vi "SetupCalc.vi"(8 "error in (no error)":errorcluster caption="entrée d'erreur (pas d'erreur)", 9 "Experiment.lvclass":refnum<class "Experiment.lvclass">=refnum, 11 "Interface en entrée":refnum<class "Interface.lvclass"> caption="Interface Class in") -> (0 "error out":errorcluster caption="sortie d'erreur", 1 "Experiment.lvclass Out":refnum<class "Experiment.lvclass">, 3 "Interface en sortie":refnum<class "Interface.lvclass"> caption="Interface Class out")   [LabVIEW 2019, in "Interface.lvclass"]
uses:
  Interface.lvclass
  Experiment Class/Experiment.lvclass
  DevicesClass/Tools/Tools.lvclass
  Calculations Class/DefaultDev_Func.ctl
  CurveSetup.ctl
  DevicesClass/BaseDevice/BaseDevice.lvclass
  Calculations Class/Calculations.lvclass
  C:/Programmes Labview/LabscanV1A/DevicesClass/BaseDevice/BaseDevice.lvclass
  Interface.lvclass/Interface.ctl
  Experiment Class/Experiment.lvclass/Experiment.ctl
  Calculations Class/Calculations.lvclass/Calculations.ctl
  DevicesClass/BaseDevice/BaseDevice.lvclass/BaseDevice.ctl
  Calculations Class/Accessor/GetOperation Name.vi
  Experiment Class/Accessor/GetLoadedTools.vi
  DevicesClass/BaseDevice/Accessor/SetClassEvent.vi
  DevicesClass/BaseDevice/Accessor/SetClassQueue.vi
  Experiment Class/Accessor/SetLoadedTools.vi
  DevicesClass/BaseDevice/Accessor/GetClassEvent.vi
  DevicesClass/BaseDevice/Accessor/GetClassQueue.vi
panel:
  out "InstrClassEventQ":T1(array[cluster])
  out "Edit Mode":bool
  out "ToolIndex":i32
  in  "Save Par":bool
  in  "EditOper":bool
  out "LoadedTools":refnum<class "BaseDevice.lvclass">[](array[class])
  in  "OperationName":string
  out "PanelViRefOut":refnum<vi>[](array[refnum])
  out "Y Values":dbl[](array[numeric])
  out "X Values":dbl[](array[numeric])
  in  "ScanDatSrc":bool[](array[boolean])
  in  "RemOper":bool
  in  "RemDataSrc":bool
  in  "Created Calc":i32(listbox) caption="Created calculation"
  in  "Data Source":i32(listbox) caption="Calculation Data Source"
  in  "AddAqData":bool
  in  "Acquired Data List":i32(listbox)
  out "2D Scan":bool
  in  "2D Plot Act":bool caption="2D Plot"
  in  "Data Only":bool
  in  "AddDataSrc":bool
  out "GraphIndex":i32
  in  "CreateOper":bool
  in  "DisplayName":string
  out "CrvParOut":T2[](array[typedef])
  out "NomDon":string[](array[string])=["RTêta;", "X&Y;"]
  out "VarParams":string[][](array[string])
  in  "ScanParam":u16(ring) caption="Scan Parameter" items=["Tools.Ind Point(Point)", "Tools_0"]
  in  "Operation":T3
  in  "stop":bool
  in  "Scan Data List":i32(listbox)
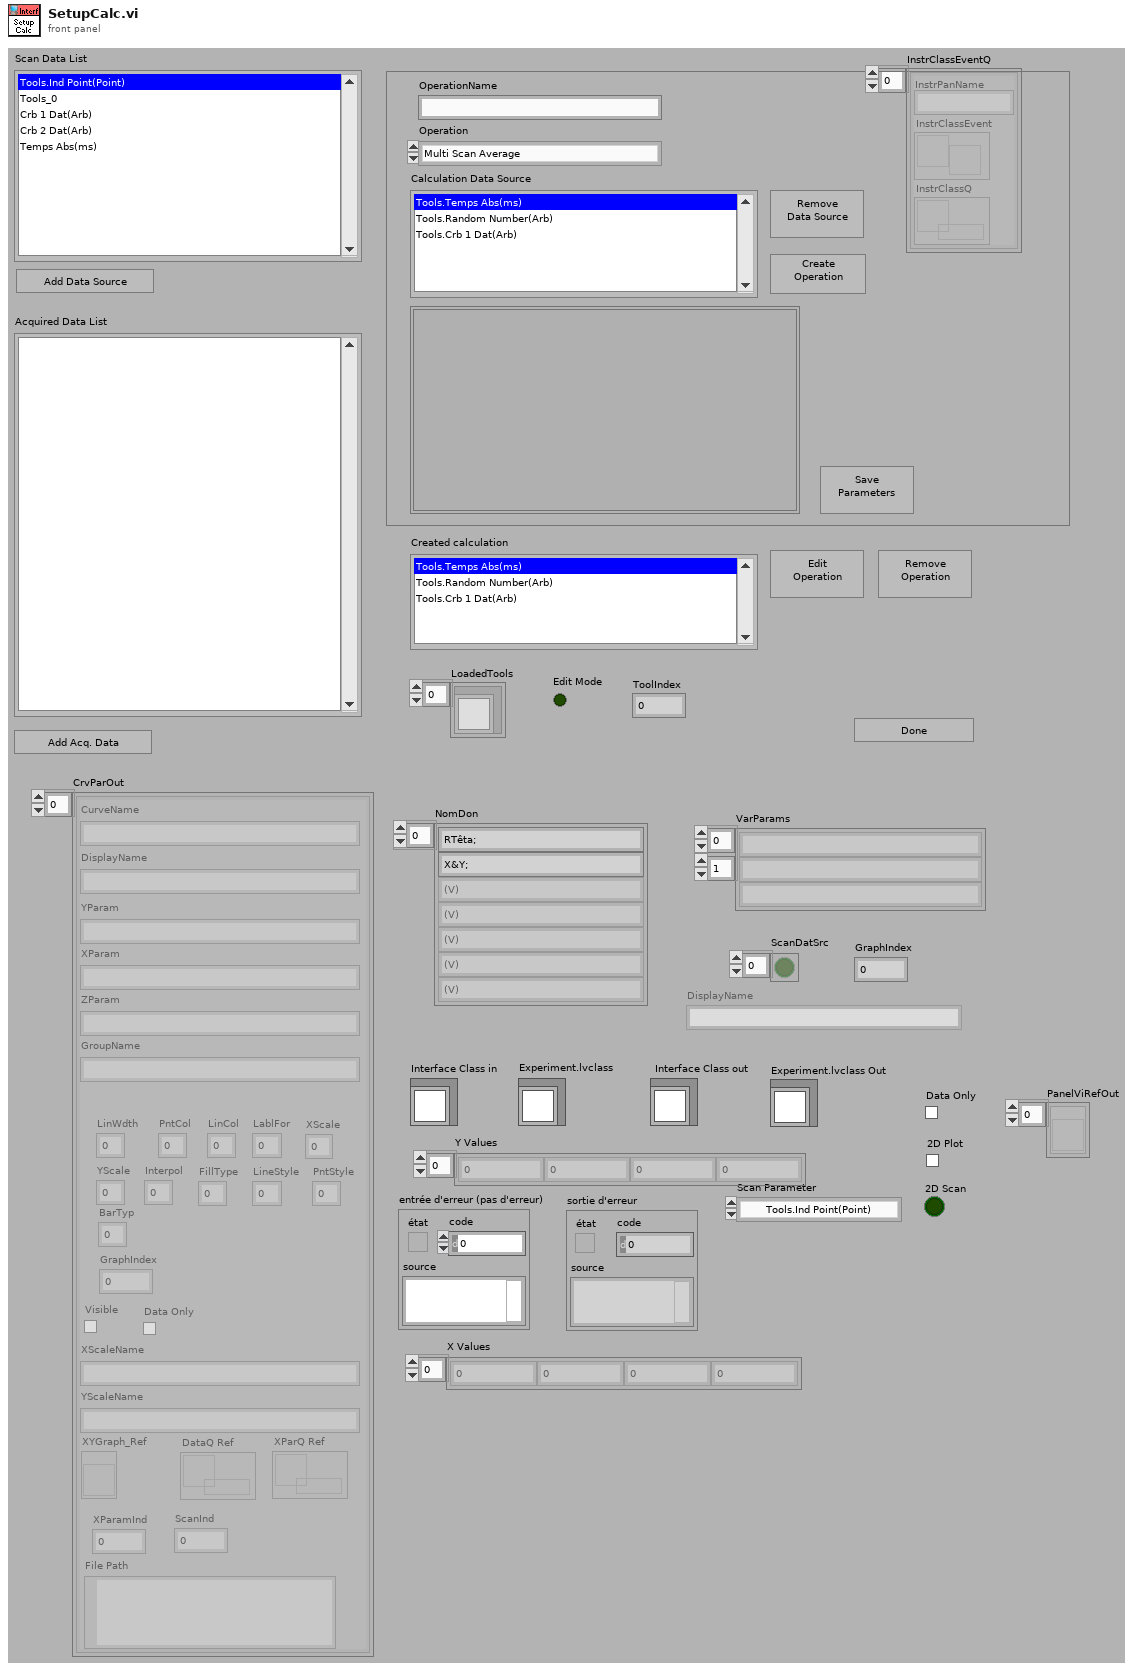
[diagram p1: front panel]
types:
  T1 = cluster{"InstrPanName":string, "InstrClassEvent":refnum<user-event>, "InstrClassQ":refnum<queue>}[]
  T2 = typedef "Interface.lvclass/CurveSetup.ctl" = cluster{"CurveName":string, "YParam":string, "XParam":string, "ZParam ":string, "GroupName":string, "LinWdth":u8, "PntCol":u32, "LinCol":u32, "LablFor":u8, "XScale":u32, "YScale":u32, "Interpol":u8, "DisplayName":string, "FillType":i16, "LineStyle":u8, "PntStyle":u8, "BarTyp":u8, "GraphIndex":i32, "Visible":bool, "XScaleName":string, "YScaleName":string, "XYGraph_Ref":refnum<vi>, "Data Only":bool, "DataQ Ref":refnum<queue>, "XParQ Ref":refnum<queue>, "XParamInd":i32, "ScanInd":i32, "File Path":path}
  T3 = typedef "Calculations.lvclass/DefaultDev_Func.ctl" = enum16{"Multi Scan Average", "Running Average", "Summ"}
  T4 = cluster{"Message":string, "Data":variant, "Code":i32}
  T5 = cluster{"InstrPanName":string, "InstrClassEvent":refnum<user-event>, "InstrClassQ":refnum<queue>}
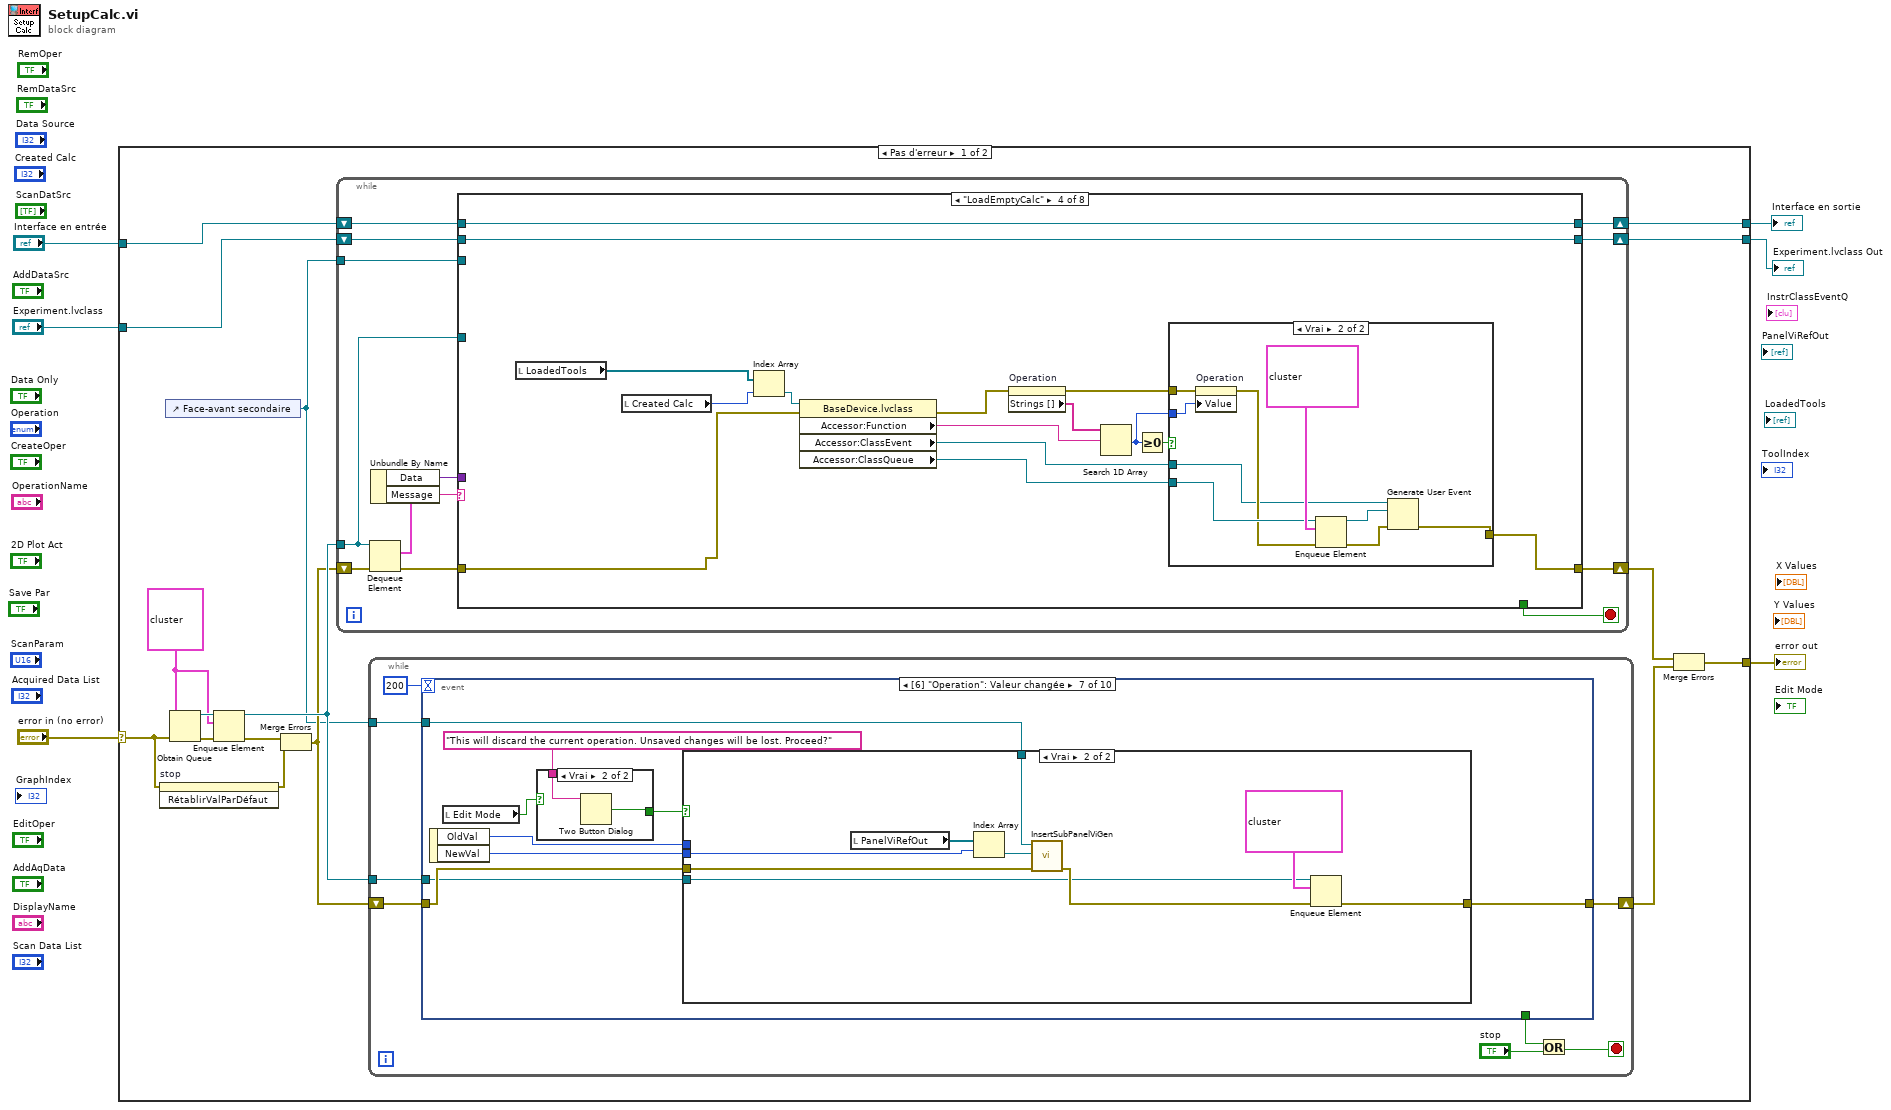
[diagram p0: block diagram]
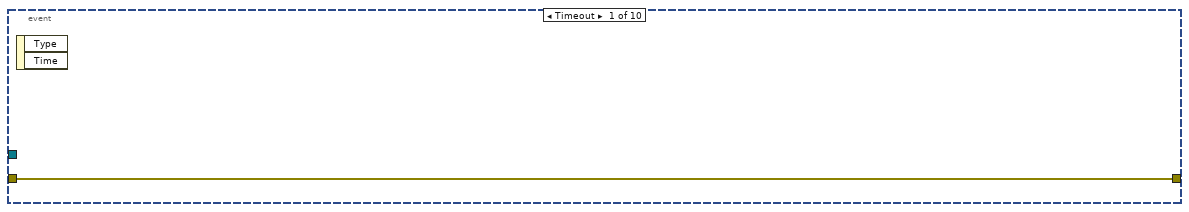
[diagram p2: hidden frame]
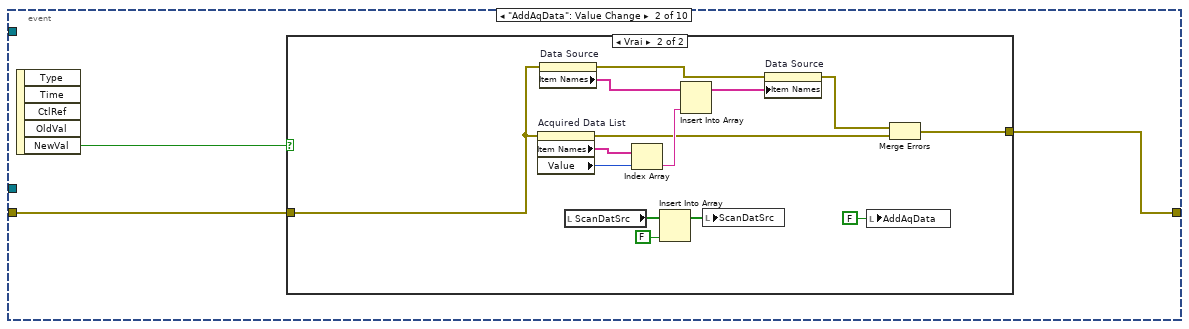
[diagram p3: hidden frame]
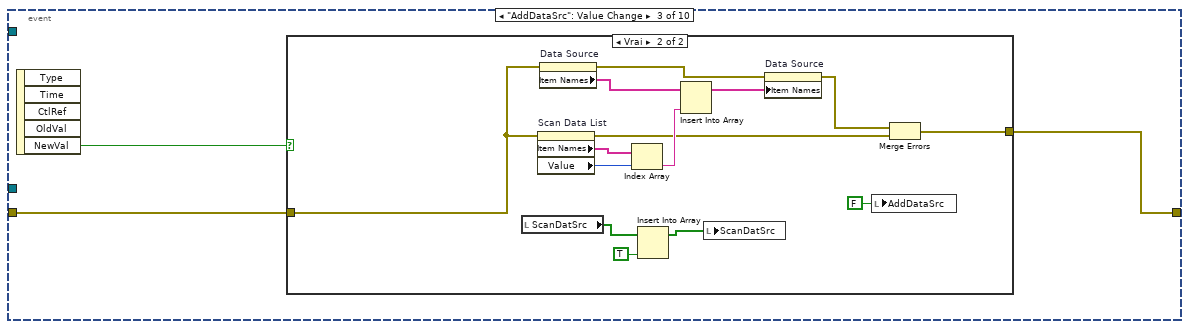
[diagram p5: hidden frame]
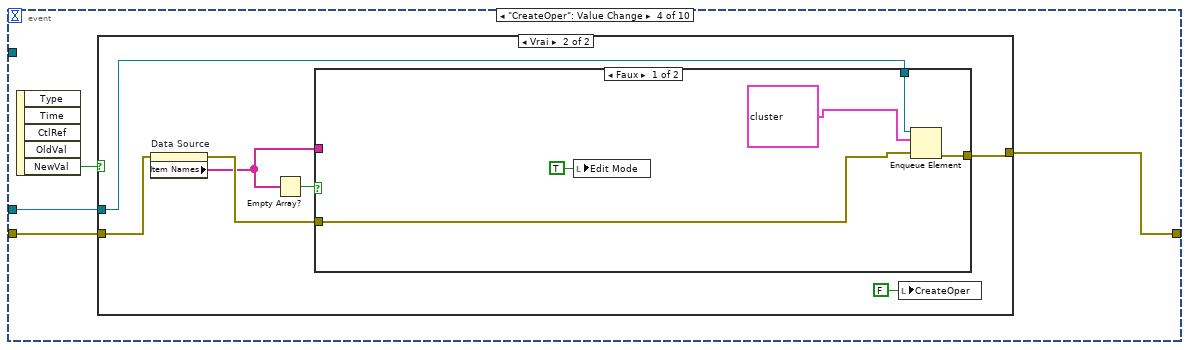
[diagram p7: hidden frame]
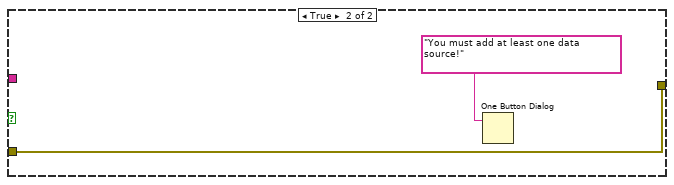
[diagram p9: hidden frame]
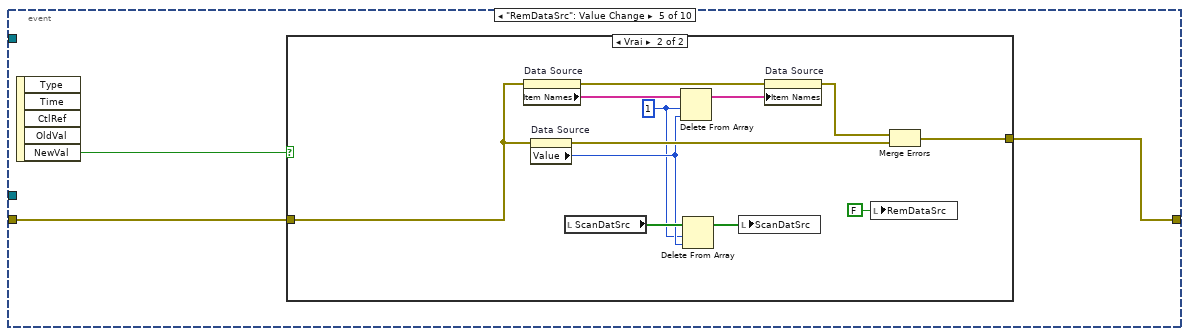
[diagram p10: hidden frame]
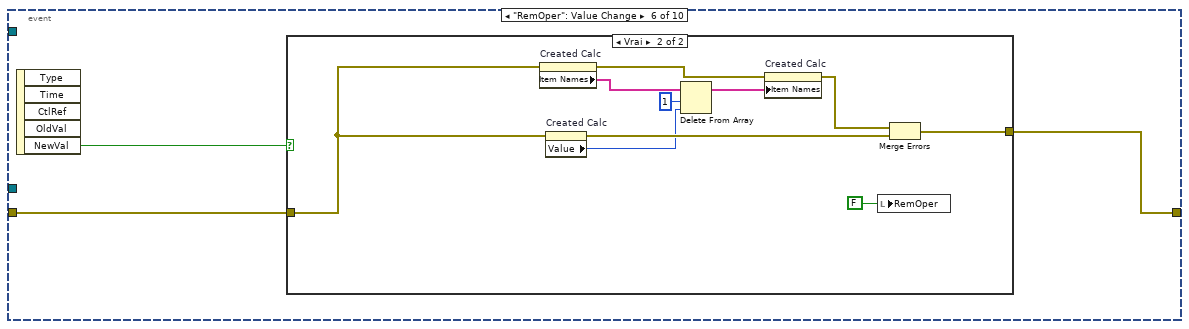
[diagram p12: hidden frame]
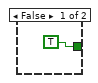
[diagram p14: hidden frame]
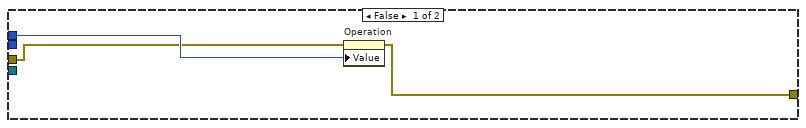
[diagram p15: hidden frame]
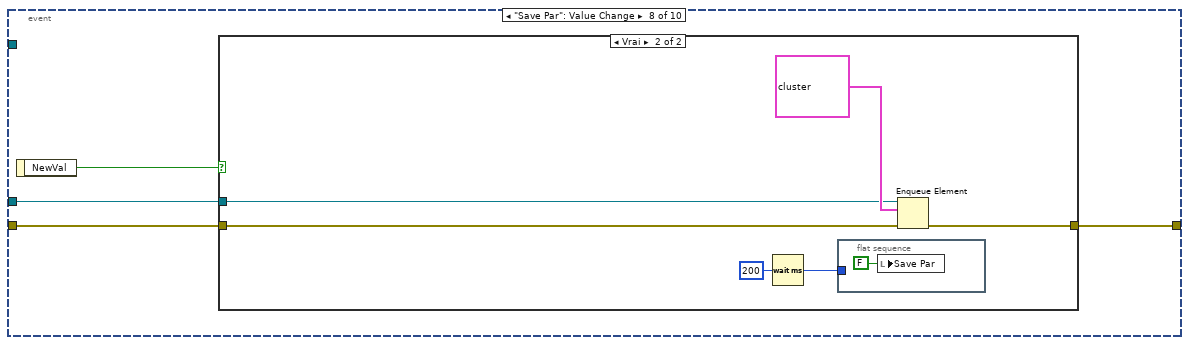
[diagram p16: hidden frame]
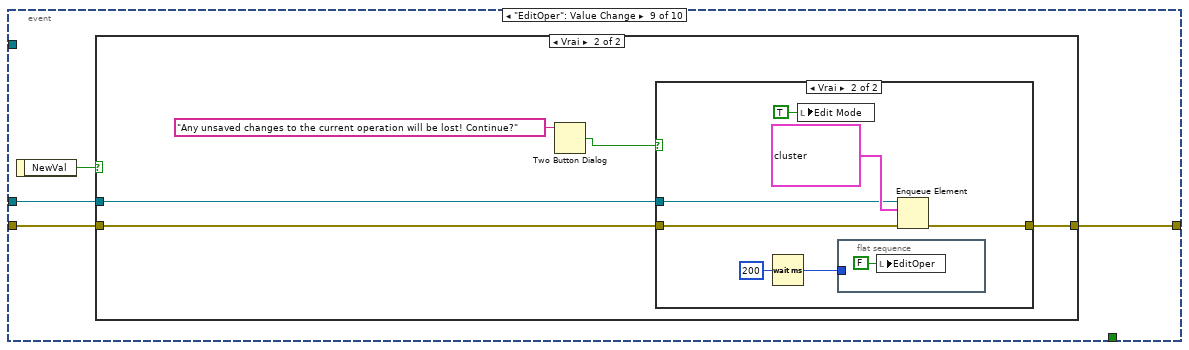
[diagram p18: hidden frame]
diagram:
  n1 = case shown="Pas d'erreur" "error in (no error)" {
    selector: "error in (no error)" -> [w18 w392]
    tunnel: [w11 w392] -> w5
    tunnel: "Interface en entrée" -> [w14 w391]
    tunnel: [w9 w391] -> w3
    tunnel: "Experiment.lvclass" -> [w19 w390]
    tunnel: [w10 w390] -> w1
    frame No Error {
      w8 = T4 {"Message"="InitProg", "Data"=variant, "Code"=0} ("Message")
      n2 = invoke on="stop" class="Bool (strict)" method="RétablirValParDéfaut"(error in=w18) -> (error out=w16:errorcluster)  [unwired: 2 in, 2 out]
      n3 = control-ref of="Face-avant secondaire"() -> (w7:refnum<vi>)
      n4 = Obtain Queue(element data type=w8, error in (no error)=w18) -> (queue out=w22:refnum<queue>, error out=w21:errorcluster)  [unwired: 3 in, 1 out]
      n5 = Enqueue Element(queue=w22, element=w8, error in (no error)=w21) -> (queue out=w20:refnum<queue>, error out=w17:errorcluster)  [unwired: 1 in, 1 out]
      n6 = Merge Errors(w17, w16) -> (w15:errorcluster)
      n7 = while {
        shift-right: [w183] -> w12
        shift-left: w15 -> [w190]
        tunnel: w20 -> [w182]
        shift-right: [w184] -> w9
        shift-left: w14 -> [w188]
        shift-right: [w186] -> w10
        shift-left: w19 -> [w189]
        tunnel: w7 -> [w181]
        stop <- w185 stop-if-true
        n8 = Dequeue Element(queue=w182, error in (no error)=w190) -> (element=w180:T4, error out=w187:errorcluster)  [unwired: 1 in, 2 out]
        n9 = Unbundle By Name(w180) -> ("Data"=w178:variant, "Message"=w179:string)
        n10 = case shown="\"LoadEmptyCalc\"" w179 {
          tunnel: w189 -> [w210 w257 w307 w338 w361 w374 w379 w388]
          tunnel: w188 -> [w194 w251 w308 w339 w362 w375 w380 w387]
          tunnel: w187 -> [w199 w254 w303 w331 w356 w365 w378 w384]
          tunnel: [w210 w256 w307 w338 w360 w374 w379 w388] -> w186
          tunnel: [FALSE _ _ _ _ _ _ TRUE] -> w185
          tunnel: [w194 w250 w308 w339 w362 w375 w380 w387] -> w184
          tunnel: [w229 w255 w304 w325 w352 w363 w376 w385] -> w183
          tunnel: w182 -> [w211 _ _ _ _ _ _ _]
          tunnel: w181 -> [w213 _ _ _ _ _ _ w381]
          tunnel: w178 -> [_ _ _ _ w358 _ _ _]
          frame "InitProg" {
            w230 = 1 ("indice")
            w218 = 0 ("Valeur (Signalisation)")
            # "2d scan"
            # "reads the available CurveSetup or get default values"
            n11 = property class="Experiment.lvclass"(reference=w210, error in=w199) -> (reference out=w209:refnum<class "Experiment.lvclass">, error out=w208:errorcluster, "Accessor:LoadedTools"=w202:refnum<class "BaseDevice.lvclass">[])
            n12 = Unbundle By Name(w194) -> ("CurvesSetup"=→"CrvParOut":T2[], "IndCourbe"=w234:i64, "AllDataQ"=w205:string[], "AllVarParQ"=w204:string[])
            n13 = for {
              tunnel: w202 -> [w248] mode=indexing
              tunnel: [w243] -> w207 mode=indexing
              tunnel: refnum<class "Calculations.lvclass"> refnum ("Calculations.lvclass") -> [w247]
              shift-right: [w244] -> _
              shift-left: w199 -> [w245]
              n14 = To More Specific Class(target class=w247, reference=w248) -> (specific class reference=w246:refnum<class "Calculations.lvclass">)  [unwired: 1 in, 1 out]
              n15 = property class="Calculations.lvclass"(reference=w246, error in=w245) -> (error out=w244:errorcluster, "Accessor:Operation Name"=w243:string)  [unwired: 1 out]
            }
            n16 = local write "LoadedTools"(w202) -> ()
            n17 = Build Array (concatenate)(w205, w204) -> (w203:string[])
            n18 = property on="Acquired Data List" class="LstDér (strict)"("Item Names"=w203) -> ()  [unwired: 2 in, 2 out]
            n19 = call "BuildInterfData.vi"("error in"=w208, "IndCourbe"=w234, "Experiment.lvclass In"=w209) -> ("error out"=w216:errorcluster, "NomDon"=→"NomDon":string[], "Scan list"=w225:string[], "VarParams"=w206:string[][])  [unwired: 1 in, 4 out]
            "VarParams" <- w206
            n20 = call <userlib>:"ArrayTo1DString.vi"("Chaîne"="", "DelArrEnd(F)"=TRUE ("DelArrEnd"), "tableau"=w206) -> ("sortie d'erreur"=w224:errorcluster, "Array Out"=w223:string[])  [unwired: 6 in, 1 out]
            n21 = Unbundle By Name(w194) -> ("Session"=w193:i32)
            n22 = call "FormatCrvNames.vi"("entrée d'erreur"=w224, "CurveNamesIn"=w223) -> ("CurveNames"=w222:string[])  [unwired: 8 in, 1 out]
            n23 = Build Array (concatenate)(w222, w225) -> (w226:string[])
            n24 = Array Size(array=w206) -> (size(s)=w233:i32[])
            n25 = property on="Scan Data List" class="LstDér (strict)"(error in=w216, "Item Names"=w226) -> (error out=w235:errorcluster)  [unwired: 1 in, 1 out]
            n26 = Index Array(array=w206, index (row)=0 ("indice (ligne)")) -> (element=w237:string[])  [unwired: 1 in]
            n27 = Index Array(array=w233, index=w230) -> (element=w231:i32)
            n28 = call "FormatCrvNames.vi"("entrée d'erreur"=w235, "CurveNamesIn"=w237) -> ("sortie d'erreur"=w212:errorcluster, "CurveNames"=w236:string[])  [unwired: 8 in]
            n29 = Greater Or Equal?(x=w231, y=w230) -> (x >= y?=→"2D Scan":bool)
            n30 = local write "Edit Mode"(FALSE ("Edit Mode")) -> ()
            n31 = property on="ScanParam" class="MDér (strict)"(error in=w212, "Strings []"=w236) -> (error out=w239:errorcluster)  [unwired: 1 in, 1 out]
            n32 = property on="Created Calc" class="LstDér (strict)"(error in=w212, "Item Names"=w207) -> (error out=w220:errorcluster)  [unwired: 1 in, 1 out]
            n33 = property on="Data Source" class="LstDér (strict)"(error in=w212, "Item Names"=string[] []) -> (error out=w221:errorcluster)  [unwired: 1 in, 1 out]
            n34 = call "LoadCalcParPanel.vi"("CalcProgQ"=w211, "error in (no error)"=w212, "Session"=w193, "RemPanRef"=w213) -> ("sortie d'erreur"=w192:errorcluster, "InstrClassEventQ"=w191:T1, "PanelViRefOut"=w201:refnum<vi>[])  [unwired: 5 in]
            n35 = local write "OperationName"("" ("OperationName")) -> ()
            n36 = property on="Scan Data List" class="LstDér (strict)"(error in=w239, "Value"=w218) -> (error out=w238:errorcluster)  [unwired: 1 in, 1 out]
            n37 = property on="Created Calc" class="LstDér (strict)"(error in=w220, "Value"=w218) -> (error out=w215:errorcluster)  [unwired: 1 in, 1 out]
            n38 = property on="Data Source" class="LstDér (strict)"(error in=w221, "Value"=w218) -> (error out=w214:errorcluster)  [unwired: 1 in, 1 out]
            n39 = local write "PanelViRefOut"(w201) -> ()
            n40 = local write "InstrClassEventQ"(w191) -> ()
            n41 = property on="Operation" class="Énum (strict)"(error in=w192, "Val(Sgnl)"=0) -> (error out=w197:errorcluster)  [unwired: 1 in, 1 out]
            n42 = Merge Errors(w197, w215, w214, w238) -> (w229:errorcluster)
          }
          frame "CreateCalc" {
            n43 = local read "ScanDatSrc"() -> (w253:bool[])
            n44 = local read "OperationName"() -> (w249:string)
            n45 = Or Array Elements(Boolean array=w253) -> (logical OR=w252:bool)
            n46 = case shown="Vrai" w252 {
              tunnel: w257 -> [w258 w274]
              tunnel: [w258 w273] -> w256
              tunnel: [w259 w272] -> w255
              tunnel: w254 -> [w260 w271]
              tunnel: w251 -> [w262 w263]
              tunnel: [w261 w263] -> w250
              tunnel: w249 -> [_ w267]
              frame False {
                n47 = call "AddCurve.vi"("error in"=w260, "InterfaceIn"=w262) -> ("error out"=w259:errorcluster, "InterfaceOut"=w261:refnum<class "Interface.lvclass">)  [unwired: 8 in]
              }
              frame True {
                # "at least one scan data source"
                n48 = property on="Created Calc" class="LstDér (strict)"(error in=w271) -> (error out=w270:errorcluster, "Item Names"=w264:string[])  [unwired: 1 in, 1 out]
                n49 = Search 1D Array(1D array=w264, element=w267) -> (index of element=w269:i32)  [unwired: 1 in]
                n50 = Greater Or Equal To 0?(x=w269) -> (x >= 0?=w268:bool)
                n51 = Empty String/Path?(string/path=w267) -> (empty?=w266:bool)
                n52 = Or(x=w266, y=w268) -> (x .or. y?=w265:bool)
                n53 = case shown="Faux" w265 {
                  tunnel: w274 -> [w279 w295]
                  tunnel: [w280 w295] -> w273
                  tunnel: [w283 w290] -> w272
                  tunnel: w270 -> [w288 w290]
                  tunnel: w267 -> [w278 _]
                  tunnel: w268 -> [_ w294]
                  tunnel: w264 -> [w286 _]
                  frame False {
                    n54 = local read "InstrClassEventQ"() -> (w277:T1)
                    n55 = local read "Operation"() -> (w276:T3)
                    n56 = property on="Data Source" class="LstDér (strict)"(error in=w288) -> (error out=w287:errorcluster, "Item Names"=w289:string[])  [unwired: 1 in, 1 out]
                    n57 = Index Array(array=w277, index=w276) -> (element=w275:T5)
                    n58 = call "LoadCalcFunc.vi"("InstrPar"=w275, "Operation Name"=w278, "ErrorIn(No Error)"=w287, "DataQNames"=w289, "Calc_Func"=w276, "Experiment.lvclass"=w279) -> ("sortie d'erreur"=w284:errorcluster, "LoadedTools"=w281:refnum<class "BaseDevice.lvclass">[], "ToolIndex"=w282:i32, "Experiment.lvclass Out"=w280:refnum<class "Experiment.lvclass">)  [unwired: 2 in]
                    n59 = Build Array (concatenate)(w286, w278) -> (w285:string[])
                    n60 = local write "LoadedTools"(w281) -> ()
                    n61 = local write "ToolIndex"(w282) -> ()
                    n62 = property on="Created Calc" class="LstDér (strict)"(error in=w284, "Item Names"=w285) -> (error out=w283:errorcluster)  [unwired: 1 in, 1 out]
                  }
                  frame True {
                    n63 = Select(t="Operation name already exist!", s=w294, f="Operation name is empty!") -> (s? t:f=w291:string)
                    n64 = One Button Dialog(message=w291) -> ()  [unwired: 1 in, 1 out]
                  }
                }
              }
            }
          }
          frame "LoadCalcOper" {
            n65 = local read "LoadedTools"() -> (w305:refnum<class "BaseDevice.lvclass">[])
            n66 = local read "Created Calc"() -> (w306:i32)
            n67 = property on="Operation" class="Énum (strict)"() -> ("Strings []"=w299:string[])  [unwired: 2 in, 2 out]
            n68 = Index Array(array=w305, index=w306) -> (element=w302:refnum<class "BaseDevice.lvclass">)
            n69 = property class="BaseDevice.lvclass"(reference=w302, error in=w303) -> (reference out=w301:refnum<class "BaseDevice.lvclass">, error out=w300:errorcluster, "Accessor:Function"=w296:string)
            n70 = Search 1D Array(1D array=w299, element=w296) -> (index of element=w297:i32)  [unwired: 1 in]
            n71 = Greater Or Equal To 0?(x=w297) -> (x >= 0?=w298:bool)
            n72 = case shown="Vrai" w298 {
              tunnel: [w309 w324] -> w304
              tunnel: w301 -> [_ w318]
              tunnel: w300 -> [w309 w317]
              tunnel: w297 -> [_ w310]
              tunnel: w296 -> [_ _]
              frame False {
              }
              frame True {
                n73 = local read "InstrClassEventQ"() -> (w322:T1)
                n74 = Index Array(array=w322, index=w310) -> (element=w321:T5)
                n75 = Unbundle By Name(w321) -> ("InstrClassEvent"=w320:refnum<user-event>, "InstrClassQ"=w319:refnum<queue>)
                n76 = property class="BaseDevice.lvclass"(reference=w318, error in=w317, "Accessor:ClassEvent"=w320, "Accessor:ClassQueue"=w319) -> (reference out=w323:refnum<class "BaseDevice.lvclass">, error out=w312:errorcluster)
                n77 = property on="Operation" class="Énum (strict)"(error in=w312, "Value"=w310) -> (error out=w311:errorcluster)  [unwired: 1 in, 1 out]
                n78 = Bundle By Name(cluster=cluster{"Message":string, "Data":variant, i32} {"Message"="SetCalcClass", "Data"=variant, 0} ("Message"), "Data"=w323) -> (w313:cluster{"Message":string, "Data":variant, i32})
                n79 = Enqueue Element(queue=w319, element=w313, error in (no error)=w311) -> (queue out=w314:refnum<queue>, error out=w315:errorcluster)  [unwired: 1 in, 1 out]
                n80 = Generate User Event(user event=w320, event data cluster=w314, error in=w315) -> (error out=w324:errorcluster)  [unwired: 1 in, 1 out]
              }
            }
          }
          frame "LoadEmptyCalc" {
            n81 = local read "LoadedTools"() -> (w336:refnum<class "BaseDevice.lvclass">[])
            n82 = local read "Created Calc"() -> (w337:i32)
            n83 = Index Array(array=w336, index=w337) -> (element=w335:refnum<class "BaseDevice.lvclass">)
            n84 = property class="BaseDevice.lvclass"(reference=w335, error in=w331) -> (error out=w333:errorcluster, "Accessor:Function"=w334:string, "Accessor:ClassEvent"=w327:refnum<user-event>, "Accessor:ClassQueue"=w326:refnum<queue>)  [unwired: 1 out]
            n85 = property on="Operation" class="Énum (strict)"(error in=w333) -> (error out=w328:errorcluster, "Strings []"=w332:string[])  [unwired: 1 in, 1 out]
            n86 = Search 1D Array(1D array=w332, element=w334) -> (index of element=w329:i32)  [unwired: 1 in]
            n87 = Greater Or Equal To 0?(x=w329) -> (x >= 0?=w330:bool)
            n88 = case shown="Vrai" w330 {
              tunnel: w329 -> [_ w349]
              tunnel: w328 -> [w340 w348]
              tunnel: w327 -> [_ w342]
              tunnel: w326 -> [_ w346]
              tunnel: [w340 w343] -> w325
              frame False {
              }
              frame True {
                n89 = property on="Operation" class="Énum (strict)"(error in=w348, "Value"=w349) -> (error out=w345:errorcluster)  [unwired: 1 in, 1 out]
                n90 = Enqueue Element(queue=w346, element=cluster{"Message":string, "Data":variant, i32} {"Message"="ResetCalcClass", "Data"=variant, 0} ("Message"), error in (no error)=w345) -> (queue out=w341:refnum<queue>, error out=w344:errorcluster)  [unwired: 1 in, 1 out]
                n91 = Generate User Event(user event=w342, event data cluster=w341, error in=w344) -> (error out=w343:errorcluster)  [unwired: 1 in, 1 out]
              }
            }
          }
          frame "CalcClassExchange" {
            n92 = Variant To Data(error in=w356, type=refnum<class "Calculations.lvclass"> refnum ("Calculations.lvclass"), Variant=w358) -> (data=w355:refnum<class "Calculations.lvclass">, error out=w353:errorcluster)
            n93 = local read "LoadedTools"() -> (w359:refnum<class "BaseDevice.lvclass">[])
            n94 = local read "ToolIndex"() -> (w354:i32)
            n95 = Replace Array Subset(array=w359, new element=w355, index=w354) -> (w351:refnum<class "BaseDevice.lvclass">[])
            n96 = local write "LoadedTools"(w351) -> ()
            n97 = property class="Experiment.lvclass"(reference=w361, error in=w353, "Accessor:LoadedTools"=w351) -> (reference out=w360:refnum<class "Experiment.lvclass">, error out=w352:errorcluster)
            n98 = local write "Edit Mode"(FALSE ("Edit Mode")) -> ()
          }
          frame "ReqCalcPar" {
            n99 = local read "LoadedTools"() -> (w373:refnum<class "BaseDevice.lvclass">[])
            n100 = local read "ToolIndex"() -> (w372:i32)
            n101 = Index Array(array=w373, index=w372) -> (element=w371:refnum<class "BaseDevice.lvclass">)
            n102 = property class="BaseDevice.lvclass"(reference=w371, error in=w365) -> (error out=w364:errorcluster, "Accessor:ClassEvent"=w368:refnum<user-event>, "Accessor:ClassQueue"=w366:refnum<queue>)  [unwired: 1 out]
            n103 = Enqueue Element(queue=w366, element=cluster{"Message":string, "Data":variant, i32} {"Message"="GetCalcClass", "Data"=variant, 0} ("Message"), error in (no error)=w364) -> (queue out=w370:refnum<queue>, error out=w369:errorcluster)  [unwired: 1 in, 1 out]
            n104 = Generate User Event(user event=w368, event data cluster=w370, error in=w369) -> (error out=w363:errorcluster)  [unwired: 1 in, 1 out]
          }
          frame "Error", Default {
            n105 = call <vilib>:"Simple Error Handler.vi"("error in (no error)"=w378) -> ("error out"=w377:errorcluster)  [unwired: 4 in, 4 out]
            n106 = call <vilib>:"Clear Errors.vi"("error in (no error)"=w377) -> ("error out"=w376:errorcluster)  [unwired: 5 in, 1 out]
          }
          frame "Stop" {
            n107 = local read "PanelViRefOut"() -> (w382:refnum<vi>[])
            n108 = call "CloseCalcPanel.vi"("error in (no error)"=w384, "SubPanRef"=w381, "PanelViRefOut"=w382) -> ("sortie d'erreur"=w383:errorcluster)  [unwired: 8 in]
            n109 = control-ref of="ce VI"() -> (w386:refnum<vi>)
            n110 = invoke class="VI" method="FA.Fermer"(reference=w386, error in=w383) -> (error out=w385:errorcluster)  [unwired: 1 in, 2 out]
          }
        }
      }
      n111 = while {
        shift-right: [w27] -> w13
        shift-left: w15 -> [w28]
        tunnel: w20 -> [w29]
        tunnel: w7 -> [w23]
        stop <- w25 stop-if-true
        n112 = event shown="[6] \"Operation\": Valeur changée" {
          selector: _ -> [_ _ _ _ _ _ _ _ _ _]
          dyn-events: _ -> [_ _ _ _ _ _ _ _ _ _]
          timeout: 200 -> [_ _ _ _ _ _ _ _ _ _]
          tunnel: w29 -> [_ _ _ w68 _ _ w121 w143 w155 w175]
          tunnel: w28 -> [w31 w33 w51 w70 w88 w104 w123 w142 w154 w177]
          tunnel: [w31 w32 w50 w69 w87 w103 w122 w144 w156 w176] -> w27
          tunnel: [_ _ _ _ _ _ _ _ _ TRUE] -> w24
          tunnel: w23 -> [_ _ _ _ _ _ w124 _ _ _]
          event Timeout {
            n113 = event-data() -> ()  [unwired: 1 in, 2 out]
          }
          event "AddAqData": Value Change {
            n114 = event-data() -> ("NewVal"=w34:bool)  [unwired: 1 in, 4 out]
            n115 = case shown="Vrai" w34 {
              tunnel: w33 -> [w35 w41]
              tunnel: [w35 w40] -> w32
              frame False {
              }
              frame True {
                n116 = property on="Acquired Data List" class="LstDér (strict)"(error in=w41) -> (error out=w42:errorcluster, "Item Names"=w49:string[], "Value"=w48:i32)  [unwired: 1 in, 1 out]
                n117 = property on="Data Source" class="LstDér (strict)"(error in=w41) -> (error out=w44:errorcluster, "Item Names"=w46:string[])  [unwired: 1 in, 1 out]
                n118 = local read "ScanDatSrc"() -> (w38:bool[])
                n119 = Index Array(array=w49, index=w48) -> (element=w47:string)
                n120 = Insert Into Array(array=w38, new element=FALSE ("new element/subarray")) -> (w37:bool[])  [unwired: 1 in]
                n121 = Insert Into Array(array=w46, new element=w47) -> (w45:string[])  [unwired: 1 in]
                n122 = local write "ScanDatSrc"(w37) -> ()
                n123 = property on="Data Source" class="LstDér (strict)"(error in=w44, "Item Names"=w45) -> (error out=w43:errorcluster)  [unwired: 1 in, 1 out]
                n124 = local write "AddAqData"(FALSE ("AddAqData")) -> ()
                n125 = Merge Errors(w43, w42) -> (w40:errorcluster)
              }
            }
          }
          event "AddDataSrc": Value Change {
            n126 = event-data() -> ("NewVal"=w52:bool)  [unwired: 1 in, 4 out]
            n127 = case shown="Vrai" w52 {
              tunnel: w51 -> [w53 w59]
              tunnel: [w53 w58] -> w50
              frame False {
              }
              frame True {
                n128 = local read "ScanDatSrc"() -> (w56:bool[])
                n129 = property on="Scan Data List" class="LstDér (strict)"(error in=w59) -> (error out=w60:errorcluster, "Item Names"=w67:string[], "Value"=w66:i32)  [unwired: 1 in, 1 out]
                n130 = property on="Data Source" class="LstDér (strict)"(error in=w59) -> (error out=w62:errorcluster, "Item Names"=w64:string[])  [unwired: 1 in, 1 out]
                n131 = Index Array(array=w67, index=w66) -> (element=w65:string)
                n132 = Insert Into Array(array=w56, new element=TRUE ("new element/subarray")) -> (w55:bool[])  [unwired: 1 in]
                n133 = Insert Into Array(array=w64, new element=w65) -> (w63:string[])  [unwired: 1 in]
                n134 = local write "ScanDatSrc"(w55) -> ()
                n135 = property on="Data Source" class="LstDér (strict)"(error in=w62, "Item Names"=w63) -> (error out=w61:errorcluster)  [unwired: 1 in, 1 out]
                n136 = local write "AddDataSrc"(FALSE ("AddDataSrc")) -> ()
                n137 = Merge Errors(w61, w60) -> (w58:errorcluster)
              }
            }
          }
          event "CreateOper": Value Change {
            n138 = event-data() -> ("NewVal"=w71:bool)  [unwired: 1 in, 4 out]
            n139 = case shown="Vrai" w71 {
              tunnel: w70 -> [w72 w78]
              tunnel: [w72 w76] -> w69
              tunnel: w68 -> [_ w75]
              frame False {
              }
              frame True {
                n140 = property on="Data Source" class="LstDér (strict)"(error in=w78) -> (error out=w79:errorcluster, "Item Names"=w73:string[])  [unwired: 1 in, 1 out]
                n141 = Empty Array?(array=w73) -> (empty?=w74:bool)
                n142 = case shown="Faux" w74 {
                  tunnel: w79 -> [w81 w86]
                  tunnel: [w84 w86] -> w76
                  tunnel: w75 -> [w83 _]
                  tunnel: w73 -> [_ _]
                  frame False {
                    n143 = local write "Edit Mode"(TRUE ("Edit Mode")) -> ()
                    n144 = Enqueue Element(queue=w83, element=cluster{"Message":string, "Data":variant, i32} {"Message"="CreateCalc", "Data"=variant, 0} ("Message"), error in (no error)=w81) -> (error out=w84:errorcluster)  [unwired: 1 in, 2 out]
                  }
                  frame True {
                    n145 = One Button Dialog(message="You must add at least one data source!") -> ()  [unwired: 1 in, 1 out]
                  }
                }
                n146 = local write "CreateOper"(FALSE ("AddDataSrc")) -> ()
              }
            }
          }
          event "RemDataSrc": Value Change {
            n147 = event-data() -> ("NewVal"=w89:bool)  [unwired: 1 in, 4 out]
            n148 = case shown="Vrai" w89 {
              tunnel: w88 -> [w90 w97]
              tunnel: [w90 w96] -> w87
              frame False {
              }
              frame True {
                w91 = 1 ("length")
                n149 = property on="Data Source" class="LstDér (strict)"(error in=w97) -> (error out=w100:errorcluster, "Item Names"=w102:string[])  [unwired: 1 in, 1 out]
                n150 = property on="Data Source" class="LstDér (strict)"(error in=w97) -> (error out=w98:errorcluster, "Value"=w92:i32)  [unwired: 1 in, 1 out]
                n151 = local read "ScanDatSrc"() -> (w94:bool[])
                n152 = Delete From Array(array=w102, length=w91, index=w92) -> (array with subset deleted=w101:string[])  [unwired: 1 out]
                n153 = Delete From Array(array=w94, length=w91, index=w92) -> (array with subset deleted=w93:bool[])  [unwired: 1 out]
                n154 = local write "ScanDatSrc"(w93) -> ()
                n155 = property on="Data Source" class="LstDér (strict)"(error in=w100, "Item Names"=w101) -> (error out=w99:errorcluster)  [unwired: 1 in, 1 out]
                n156 = local write "RemDataSrc"(FALSE ("AddDataSrc")) -> ()
                n157 = Merge Errors(w99, w98) -> (w96:errorcluster)
              }
            }
          }
          event "RemOper": Value Change {
            n158 = event-data() -> ("NewVal"=w105:bool)  [unwired: 1 in, 4 out]
            n159 = case shown="Vrai" w105 {
              tunnel: w104 -> [w106 w111]
              tunnel: [w106 w110] -> w103
              frame False {
              }
              frame True {
                n160 = property on="Created Calc" class="LstDér (strict)"(error in=w111) -> (error out=w114:errorcluster, "Item Names"=w116:string[])  [unwired: 1 in, 1 out]
                n161 = property on="Created Calc" class="LstDér (strict)"(error in=w111) -> (error out=w112:errorcluster, "Value"=w108:i32)  [unwired: 1 in, 1 out]
                n162 = Delete From Array(array=w116, length=1, index=w108) -> (array with subset deleted=w115:string[])  [unwired: 1 out]
                n163 = property on="Created Calc" class="LstDér (strict)"(error in=w114, "Item Names"=w115) -> (error out=w113:errorcluster)  [unwired: 1 in, 1 out]
                n164 = local write "RemOper"(FALSE ("AddDataSrc")) -> ()
                n165 = Merge Errors(w113, w112) -> (w110:errorcluster)
              }
            }
          }
          event Value Change {
            n166 = event-data() -> ("OldVal"=w117:T3, "NewVal"=w125:T3)  [unwired: 1 in]
            n167 = local read "Edit Mode"() -> (w120:bool)
            n168 = case shown="Vrai" w120 {
              tunnel: "This will discard the current operation. Unsaved changes will be lost. Proceed?" -> [_ w128]
              tunnel: [TRUE w127] -> w118
              frame False {
              }
              frame True {
                n169 = Two Button Dialog(message=w128) -> (T button?=w127:bool)  [unwired: 2 in]
              }
            }
            n170 = case shown="Vrai" w118 {
              tunnel: w125 -> [_ w139]
              tunnel: w124 -> [_ w138]
              tunnel: w123 -> [w130 w136]
              tunnel: [w129 w134] -> w122
              tunnel: w121 -> [_ w132]
              tunnel: w117 -> [w131 _]
              frame False {
                n171 = property on="Operation" class="Énum (strict)"(error in=w130, "Value"=w131) -> (error out=w129:errorcluster)  [unwired: 1 in, 1 out]
              }
              frame True {
                n172 = local read "PanelViRefOut"() -> (w140:refnum<vi>[])
                n173 = Index Array(array=w140, index=w139) -> (element=w137:refnum<vi>)
                n174 = call <userlib>:"InsertSubPanelViGen.vi"("error in (no error)"=w136, "RemVIRef"=w137, "RemPanRef"=w138) -> ("sortie d'erreur"=w135:errorcluster)  [unwired: 6 in, 2 out]
                n175 = Enqueue Element(queue=w132, element=cluster{"Message":string, "Data":variant, i32} {"Message"="LoadEmptyCalc", "Data"=variant, 0} ("Message"), error in (no error)=w135) -> (error out=w134:errorcluster)  [unwired: 1 in, 2 out]
              }
            }
          }
          event "Save Par": Value Change {
            n176 = event-data() -> ("NewVal"=w141:bool)  [unwired: 1 in]
            n177 = case shown="Vrai" w141 {
              tunnel: [w145 w151] -> w144
              tunnel: w143 -> [_ w149]
              tunnel: w142 -> [w145 w148]
              frame False {
              }
              frame True {
                n178 = Wait (ms)(milliseconds to wait=u32 200 ("attente (ms)")) -> (millisecond timer value=w147:u32)
                n179 = flat-sequence {
                  tunnel: w147 -> [_]
                  frame #0 {
                    n180 = local write "Save Par"(FALSE ("Save Par")) -> ()
                  }
                }
                n181 = Enqueue Element(queue=w149, element=cluster{"Message":string, "Data":variant, i32} {"Message"="ReqCalcPar", "Data"=variant, 0} ("Message"), error in (no error)=w148) -> (error out=w151:errorcluster)  [unwired: 1 in, 2 out]
              }
            }
          }
          event "EditOper": Value Change {
            n182 = event-data() -> ("NewVal"=w153:bool)  [unwired: 1 in]
            n183 = case shown="Vrai" w153 {
              tunnel: [w157 w162] -> w156
              tunnel: w155 -> [_ w161]
              tunnel: w154 -> [w157 w160]
              frame False {
              }
              frame True {
                n184 = Two Button Dialog(message="Any unsaved changes to the current operation will be lost! Continue?") -> (T button?=w159:bool)  [unwired: 2 in]
                n185 = case shown="Vrai" w159 {
                  tunnel: [w163 w170] -> w162
                  tunnel: w161 -> [_ w168]
                  tunnel: w160 -> [w163 w167]
                  frame False {
                  }
                  frame True {
                    n186 = Wait (ms)(milliseconds to wait=u32 200 ("attente (ms)")) -> (millisecond timer value=w166:u32)
                    n187 = local write "Edit Mode"(TRUE ("Edit Mode")) -> ()
                    n188 = flat-sequence {
                      tunnel: w166 -> [_]
                      frame #0 {
                        n189 = local write "EditOper"(FALSE ("Save Par")) -> ()
                      }
                    }
                    n190 = Enqueue Element(queue=w168, element=cluster{"Message":string, "Data":variant, i32} {"Message"="LoadCalcOper", "Data"=variant, 0} ("Message"), error in (no error)=w167) -> (error out=w170:errorcluster)  [unwired: 1 in, 2 out]
                  }
                }
              }
            }
          }
          event "stop": Value Change; Panel Close {
            n191 = event-data() -> ()  [unwired: 1 in, 2 out]
            n192 = Enqueue Element(queue=w175, element=cluster{"Message":string, "Data":variant, i32} {"Message"="Stop", "Data"=variant, 0} ("Message"), error in (no error)=w177) -> (error out=w176:errorcluster)  [unwired: 1 in, 2 out]
            n193 = local write "stop"(FALSE ("stop")) -> ()
          }
        }
        n194 = Or(x=w24, y="stop") -> (x .or. y?=w25:bool)
      }
      n195 = Merge Errors(w12, w13) -> (w11:errorcluster)
    }
    frame Error {
    }
  }
  "error out" <- w5
  "Interface en sortie" <- w3
  "Experiment.lvclass Out" <- w1
